vi "Load Images From File.vi"(10 "Input Image Dark":T1, 11 "Input Image Light":T1) -> (2 "Dark Image Out":T1, 3 "Light Image Out":T1)   [LabVIEW 2012]
uses:
  <vilib>/vision/Image Controls.llb/IMAQ Image.ctl
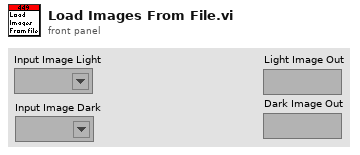
[diagram p1: front panel]
types:
  T1 = typedef "IMAQ Image.ctl" = refnum<image>
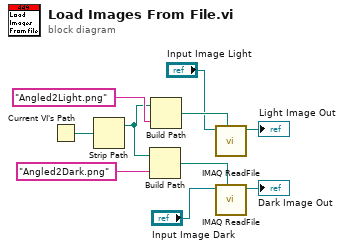
[diagram p0: block diagram]
diagram:
  n1 = Current VI's Path() -> (path=w10:path)
  n2 = Strip Path(path=w10) -> (stripped path=w8:path)  [unwired: 1 out]
  n3 = Build Path(base path=w8, name or relative path="Angled2Dark.png") -> (appended path=w3:path)
  n4 = Build Path(base path=w8, name or relative path="Angled2Light.png") -> (appended path=w6:path)
  n5 = call "IMAQ ReadFile"("File Path"=w6, "Image"="Input Image Light") -> ("Image Out"=→"Light Image Out":T1)  [unwired: 5 in, 4 out]
  n6 = call "IMAQ ReadFile"("File Path"=w3, "Image"="Input Image Dark") -> ("Image Out"=→"Dark Image Out":T1)  [unwired: 5 in, 4 out]
